vi "Auto Start.vi"(8 "error in (no error)":errorcluster, 11 "IP Address DUT X":string="localhost") -> (0 "error out":errorcluster, 3 "TCPHandle":refnum<k5>)   [LabVIEW 2012]
uses:
  Remote Sever SubVIs/TypeDef/Send Command Message.ctl
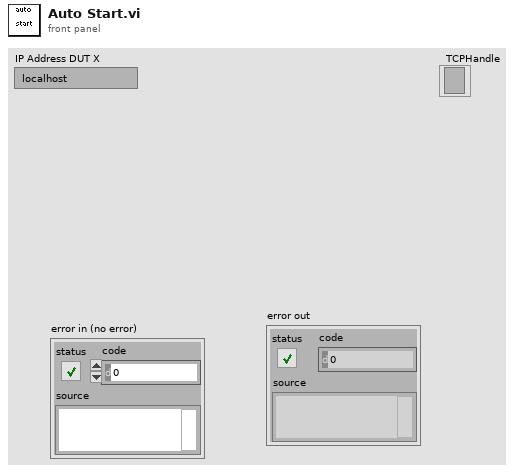
[diagram p1: front panel]
types:
  T1 = typedef "Send Command Message.ctl" = string
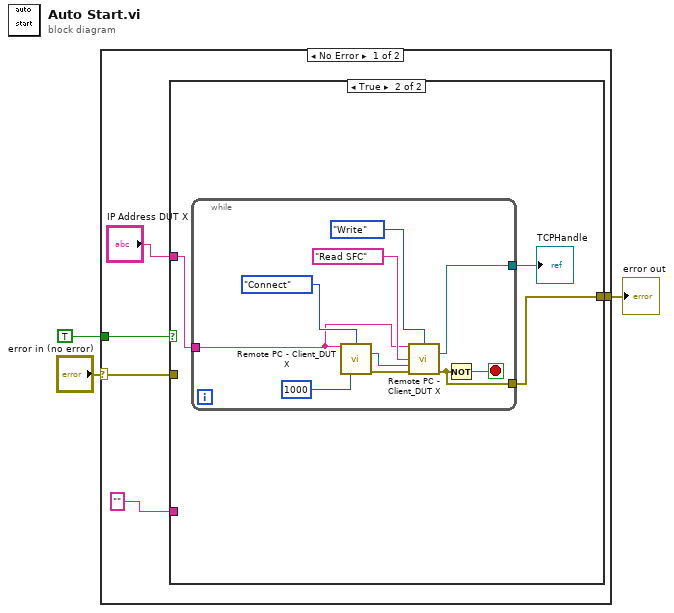
[diagram p0: block diagram]
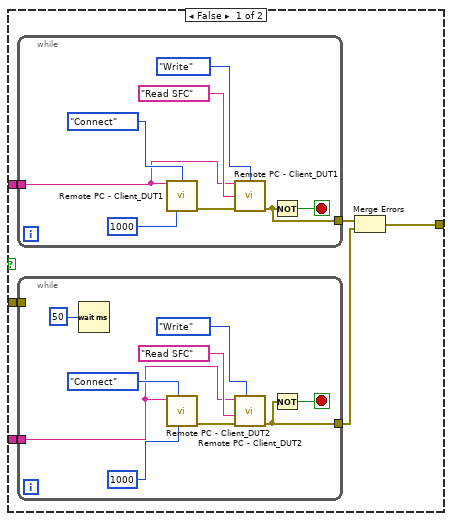
[diagram p2: hidden frame]
diagram:
  n1 = case shown="No Error" "error in (no error)" {
    selector: "error in (no error)" -> [w8 w45]
    tunnel: [w7 w45] -> w2
    tunnel: TRUE -> [w6 _]
    frame No Error {
      n2 = case shown="True" w6 {
        tunnel: w8 -> [w14 _]
        tunnel: [w12 w34] -> w7
        tunnel: "IP Address DUT X" -> [w10 w33]
        tunnel: "" ("IP Address DUT2") -> [w9 _]
        frame False {
          n3 = while {
            tunnel: [w16] -> w11
            tunnel: w10 -> [w15]
            stop <- w17 stop-if-true
            n4 = call "Remote PC - Client_DUT1.vi"("IP Address"=w15, "Flow Contorl"=enum16{"Connect", "Read", "Write", "Close"}."Connect", "Remote Sever Port (2800)"=u16 1000) -> ("error out"=w18:errorcluster)  [unwired: 9 in, 3 out]
            n5 = call "Remote PC - Client_DUT1.vi"("IP Address"=w15, "Flow Contorl"=enum16{"Connect", "Read", "Write", "Close"}."Write", "Send Command"=T1 "Read SFC", "error in"=w18) -> ("error out"=w16:errorcluster)  [unwired: 8 in, 3 out]
            n6 = Not(x=w16) -> (.not. x?=w17:bool)
          }
          n7 = while {
            tunnel: w14 -> [_]
            tunnel: [w24] -> w13
            tunnel: w9 -> [w23]
            stop <- w29 stop-if-true
            n8 = Wait (ms)(milliseconds to wait=u32 50) -> ()  [unwired: 1 out]
            n9 = call "Remote PC - Client_DUT2.vi"("Remote Sever Port (2800)"=u16 1000, "Flow Contorl"=enum16{"Connect", "Read", "Write", "Close"}."Connect", "IP Address"=w23) -> ("error out"=w27:errorcluster)  [unwired: 6 in, 2 out]
            n10 = call "Remote PC - Client_DUT2.vi"("Flow Contorl"=enum16{"Connect", "Read", "Write", "Close"}."Write", "error in"=w27, "Send Command"=T1 "Read SFC", "IP Address"=w23) -> ("error out"=w24:errorcluster)  [unwired: 5 in, 2 out]
            n11 = Not(x=w24) -> (.not. x?=w29:bool)
          }
          n12 = Merge Errors(w11, w13) -> (w12:errorcluster)
        }
        frame True {
          n13 = while {
            tunnel: [w38] -> w34
            tunnel: w33 -> [w37]
            tunnel: [w35] -> w32
            stop <- w39 stop-if-true
            n14 = call "Remote PC - Client_DUT X.vi"("IP Address"=w37, "Flow Contorl"=enum16{"Connect", "Read", "Write", "Close"}."Connect", "Remote Sever Port (2800)"=u16 1000) -> ("TCPHandle"=w36:refnum<k5>, "error out"=w40:errorcluster)  [unwired: 9 in, 2 out]
            n15 = call "Remote PC - Client_DUT X.vi"("IP Address"=w37, "Flow Contorl"=enum16{"Connect", "Read", "Write", "Close"}."Write", "Send Command"=T1 "Read SFC", "ServerTCPhandle"=w36, "error in"=w40) -> ("TCPHandle"=w35:refnum<k5>, "error out"=w38:errorcluster)  [unwired: 7 in, 2 out]
            n16 = Not(x=w38) -> (.not. x?=w39:bool)
          }
          "TCPHandle" <- w32
        }
      }
    }
    frame Error {
    }
  }
  "error out" <- w2
